vi "Save Column Widths.vi"(7 "error in":errorcluster, 9 "Display State in":T1, 10 "MCListbox Refnum in":refnum<vi>) -> (0 "error out":errorcluster, 2 "Display State out":T1, 3 "MCListbox Refnum out":refnum<vi>)   [LabVIEW 2012, in "ListBox_XControl.xctl"]
doc: "Get Column widths after resizing (to save column width state)"
uses:
  ListBox_XControl.xctl
  ListBox_State.ctl
  Order Type Def.ctl
  Value Filters.ctl
  <vilib>/Utility/miscctls.llb/LVRowAndColumnTypeDef.ctl
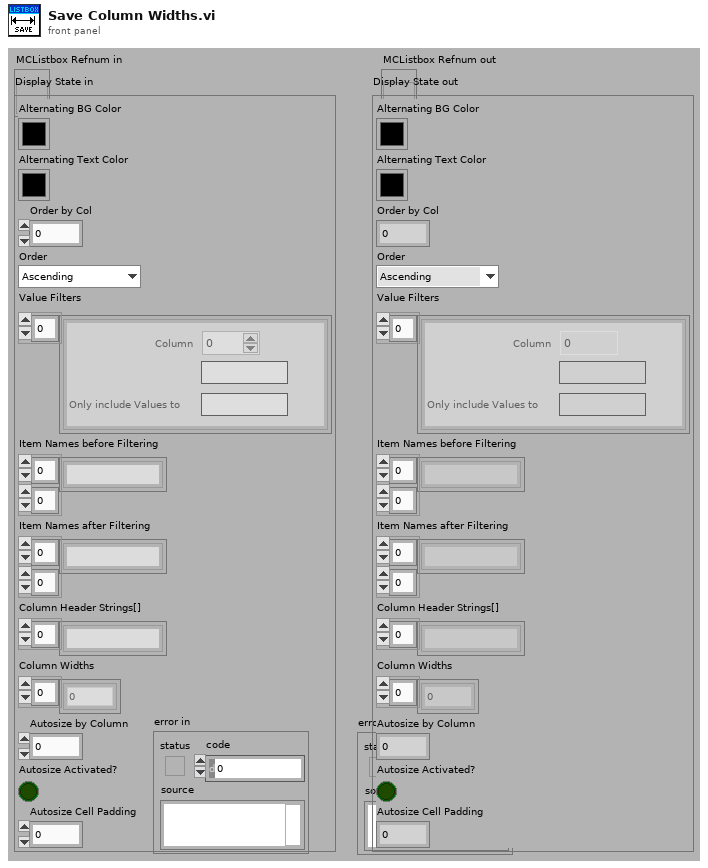
[diagram p1: front panel]
types:
  T1 = typedef "ListBox_XControl.xctl/ListBox_State.ctl" = cluster{"Alternating BG Color":u32, "Alternating Text Color":u32, "Order by Col":i32, "Order":T2, "Value Filters":T3, "Item Names before Filtering":string[][], "Item Names after Filtering":string[][], "Column Header Strings[]":string[], "Column Widths":u32[], "Autosize by Column":i32, "Autosize Activated?":bool, "Autosize Cell Padding":u32}
  T2 = typedef "ListBox_XControl.xctl/Order Type Def.ctl" = enum16{"Ascending", "Descending", "Off"}
  T3 = typedef "ListBox_XControl.xctl/Value Filters.ctl" = cluster{"Column":i32, "Only include Values From":string, "Only include Values to":string}[]
  T4 = typedef "LVRowAndColumnTypeDef.ctl" = cluster{"Row":i32, "Column":i32}
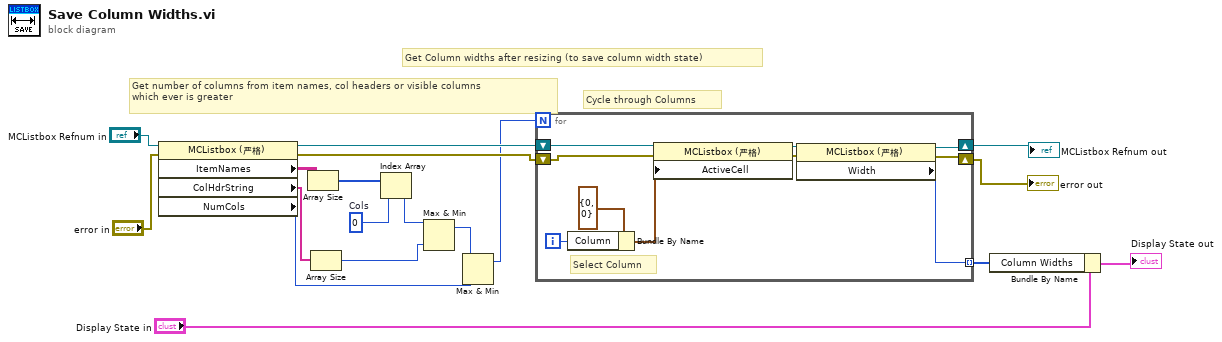
[diagram p0: block diagram]
diagram:
  w11 = 0  # Cols
  # "Get Column widths after resizing (to save column width state)"
  # "Get number of columns from item names, col headers or visible columns\nwhich ever is greater"
  # "Cycle through Columns"
  n1 = property on="Property Node" class="MCListbox (严格)"(reference="MCListbox Refnum in", error in="error in") -> (reference out=w8:refnum<vi>, error out=w6:errorcluster, "ItemNames"=w14:string[][], "ColHdrString"=w13:string[], "NumCols"=w4:u32)
  n2 = Array Size(array=w14) -> (size(s)=w12:i32[])
  n3 = Array Size(array=w13) -> (size(s)=w9:i32)
  n4 = Index Array(array=w12, index=w11) -> (element=w10:i32)
  n5 = Max & Min(x=w10, y=w9) -> (max(x,y)=w5:i32)  [unwired: 1 out]
  n6 = Max & Min(x=w5, y=w4) -> (max(x,y)=w3:u32)  [unwired: 1 out]
  n7 = for {
    N: w3 -> [_]
    shift-right: [w20] -> w2
    shift-left: w6 -> [w25]
    shift-right: [w19] -> w7
    shift-left: w8 -> [w24]
    tunnel: [w21] -> w1 mode=indexing
    i -> [w28]
    # "Select Column"
    n8 = Bundle By Name(cluster=T4 {"Row"=0, "Column"=0} ("Active Cell:Active Cell"), "Column"=w28) -> (w26:T4)
    n9 = property on="Property Node" class="MCListbox (严格)"(reference=w24, error in=w25, "ActiveCell"=w26) -> (reference out=w23:refnum<vi>, error out=w22:errorcluster)
    n10 = property on="Property Node" class="MCListbox (严格)"(reference=w23, error in=w22) -> (reference out=w19:refnum<vi>, error out=w20:errorcluster, "Width"=w21:u32)
  }
  "error out" <- w2
  "MCListbox Refnum out" <- w7
  n11 = Bundle By Name(cluster="Display State in", "Column Widths"=w1) -> (→"Display State out":T1)
